vi "Spectrogram.vi"() -> ()   [LabVIEW 2011]
uses:
  <vilib>/Analysis/4window.llb/windowTd.ctl
  <vilib>/Analysis/Matrix/Datatypes/RealMatrix.ctl
  <vilib>/Utility/file.llb/Read From Spreadsheet File (DBL).vi
  <vilib>/addons/Time Frequency Analysis/Spectrogram.llb/TFA STFT Spectrogram (Real).vi
  <vilib>/addons/_Advanced Signal Processing/NI_AdvSigProcTFA.lvlib
  <vilib>/Analysis/Matrix/NI_Matrix.lvlib
  <vilib>/Analysis/NI_AALPro.lvlib
panel:
  in  "Offset":dbl[](array[numeric])
  in  "Open":bool
  in  "Exit":bool
  in  "Sensor #":i32(ring)=2 items=["Sensor 1", "Sensor 2", "Sensor 3"]
  in  "Scan Step (mm)":dbl=0.01
  in  "Spectrogram":bool
  out "MagneScale Sensors":dbl[][](graph) caption="A - Scan Graph"
  out "STFT Spectrogram":dbl[][](graph)
  in  "window info":cluster{"type":T1, "length":i32}={"type"=62, "length"=32} {"type" items=["Rectangle"=0, "Hanning"=1, "Hamming"=2, "Blackman-Harris"=3, "Exact Blackman"=4, "Blackman"=5, "Flat Top"=6, "4 Term B-Harris "=7, "7 Term B-Harris"=8, "Low Sidelobe"=9, "Blackman Nuttall"=11, "Triangle"=30, "Bartlett-Hanning"=31, "Bohman"=32, "Parzen"=33, "Welch"=34, "Kaiser"=60, "Dolph-Chebyshev"=61, "Gaussian"=62]}
  in  "time-freq info":cluster{"time steps":i32, "frequency bins":i32}={"time steps"=1, "frequency bins"=512}
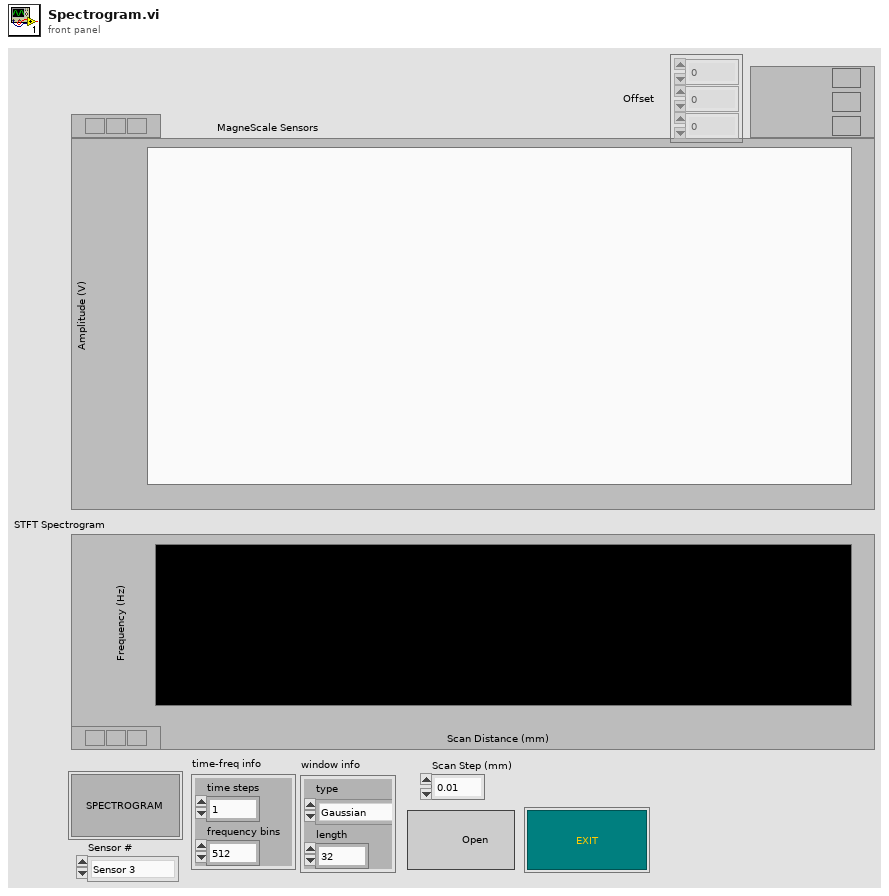
[diagram p1: front panel]
types:
  T1 = typedef "NI_AALPro.lvlib/windowTd.ctl" = u32
  T2 = typedef "NI_Matrix.lvlib/RealMatrix.ctl" = dbl[][]
  T3 = cluster{"frequency offset":dbl, "frequency multiplier":dbl}
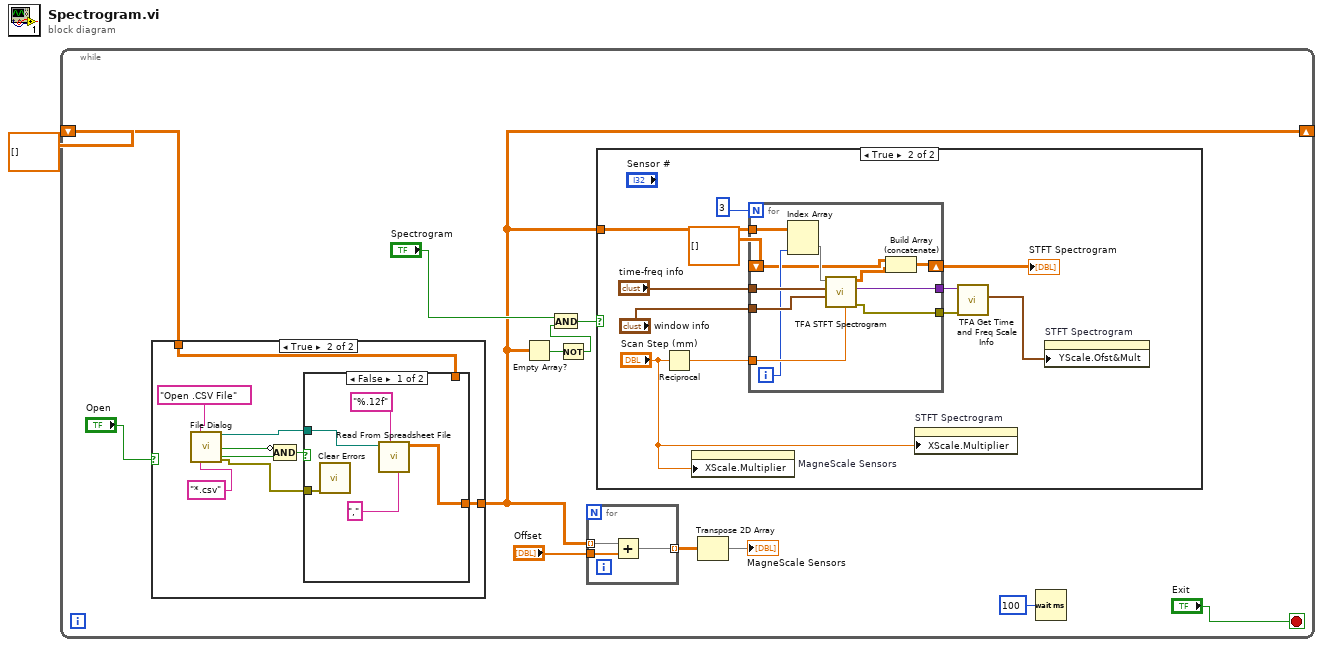
[diagram p0: block diagram]
diagram:
  n1 = while {
    shift-right: [w2] -> _
    shift-left: dbl[][] [] ("all rows") -> [w12]
    stop <- "Exit" stop-if-true
    n2 = case shown="True" "Open" {
      tunnel: [w39 w41] -> w2
      tunnel: w12 -> [w39 w40]
      frame False {
      }
      frame True {
        n3 = call "File Dialog"("prompt"="Open .CSV File" ("button label"), "pattern (all files)"="*.csv") -> ("selected path"=w48:path, "exists"=w46:bool, "cancelled"=w45:bool, "error out"=w43:errorcluster)  [unwired: 10 in]
        n4 = Compound Arithmetic op=AND(invert w46, w45) -> (w44:bool)
        n5 = case shown="False" w44 {
          tunnel: w48 -> [w51 _]
          tunnel: [w49 w54] -> w41
          tunnel: w43 -> [w50 _]
          tunnel: w40 -> [_ w54]
          frame False {
            n6 = call <vilib>:"Clear Errors.vi"("error in (no error)"=w50) -> ()  [unwired: 6 in, 1 out]
            n7 = call-poly <vilib>:"Read From Spreadsheet File.vi"("delimiter (\\t)"="," ("delimiter (\\t)"), "format (%.3f)"="%.12f", "file path (dialog if empty)"=w51) -> ("all rows"=w49:dbl[][])  [unwired: 4 in, 4 out]
          }
          frame True {
          }
        }
      }
    }
    n8 = Empty Array?(array=w2) -> (empty?=w9:bool)
    n9 = Not(x=w9) -> (.not. x?=w8:bool)
    n10 = And(x="Spectrogram", y=w8) -> (x .and. y?=w10:bool)
    n11 = for {
      tunnel: w2 -> [w16] mode=indexing
      tunnel: "Offset" -> [w15]
      tunnel: [w14] -> w4 mode=indexing
      n12 = Add(x=w16, y=w15) -> (x+y=w14:dbl[])
    }
    n13 = case shown="True" w10 {
      tunnel: w2 -> [_ w26]
      frame False {
      }
      frame True {
        n14 = Reciprocal(x="Scan Step (mm)") -> (1/x=w23:dbl)
        n15 = property on="MagneScale Sensors" class="WFGraph (strict)"("XScale.Multiplier"="Scan Step (mm)") -> ()  [unwired: 2 in, 2 out]
        n16 = for {
          N: 3 -> [_]
          tunnel: w26 -> [w38]
          tunnel: [w37] -> w25
          tunnel: [w36] -> w24
          tunnel: w23 -> [w35]
          tunnel: "time-freq info" -> [w33]
          tunnel: "window info" -> [w32]
          shift-right: [w29] -> w18
          shift-left: T2 [] ("Real Matrix") -> [w28]
          i -> [w31]
          n17 = Index Array(array=w38, index (col)=w31) -> (element=w34:dbl[])  [unwired: 1 in]
          n18 = call-poly <vilib>:"TFA STFT Spectrogram.vi"("sampling rate"=w35, "window info"=w32, "time-frequency sampling info"=w33, "signal"=w34) -> ("error out"=w37:errorcluster, "scale info"=w36:variant, "spectrogram"=w30:dbl[][])  [unwired: 5 in]
          n19 = Build Array (concatenate)(w28, w30) -> (w29:T2)
        }
        "STFT Spectrogram" <- w18
        n20 = property on="STFT Spectrogram" class="IntGraph (strict)"("XScale.Multiplier"="Scan Step (mm)") -> ()  [unwired: 2 in, 2 out]
        n21 = call <vilib>:"TFA Get Time and Freq Scale Info.vi"("error in (no error)"=w25, "scale info"=w24) -> ("frequency info"=w27:T3)  [unwired: 7 in, 2 out]
        n22 = property on="STFT Spectrogram" class="IntGraph (strict)"("YScale.Ofst&Mult"=w27) -> ()  [unwired: 2 in, 2 out]
      }
    }
    n23 = Transpose 2D Array(2D array=w4) -> (transposed array=→"MagneScale Sensors":dbl[][])
    n24 = Wait (ms)(milliseconds to wait=u32 100 ("millisecond multiple")) -> ()  [unwired: 1 out]
  }
